vi "ProcessManager.vi"() -> ()   [LabVIEW 2019]
doc: "Fonction :\n\nCe modèle peut être intégré très facilement à un subpannel à l'aide des fonctions de la palette Code Template >> Dynamic VI and Subpanel de la VIBOX"
panel:
  out "data":string[][](array[string])=[["1", "芯轴分总成磨合台"], ["2", "上管柱组件装配"], ["3", "上管柱上转向轴合成"], ["4", "滑移力检测"], ["5", "芯轴分总成NVH"], ["6", "上转向轴组件装配"], ["7", "上下管柱总成装配"], ["8", "滑移力复检"], ["9", "最终性能试验台"], ["10", "传感器对中台"], ["11", "电机装配"], ["12", "中间轴装配"], ["13", "GP12（340）"], ["14", "ECU装配"], ["22", "激光打标机"], ["26", "调节机构检测"], ["29", "调节机构装配"]]
  out "ALL_DEVICE":string[](array[string])=["芯轴分总成磨合台", "上管柱组件装配", "上管柱上转向轴合成", "滑移力检测", "芯轴分总成NVH", "上转向轴组件装配", "上下管柱总成装配", "滑移力复检", "最终性能试验台", "传感器对中台", "电机装配", "中间轴装配", "GP12（340）", "ECU装配", "激光打标机", "调节机构检测", "调节机构装配"]
  out "Stop<user event>":refnum<user-event>
  in  "保存按钮":bool
  in  "产品型号":u16(ring) caption="Enum 3" items=[""=0, "R092B"=8, "R128"=1, "R527"=4, "R538"=5, "R563A"=9, "R563X"=7, "R567X"=6, "R92A"=3]
  in  "工位名称":i32(listbox)
  in  "产品工艺":string(tree)
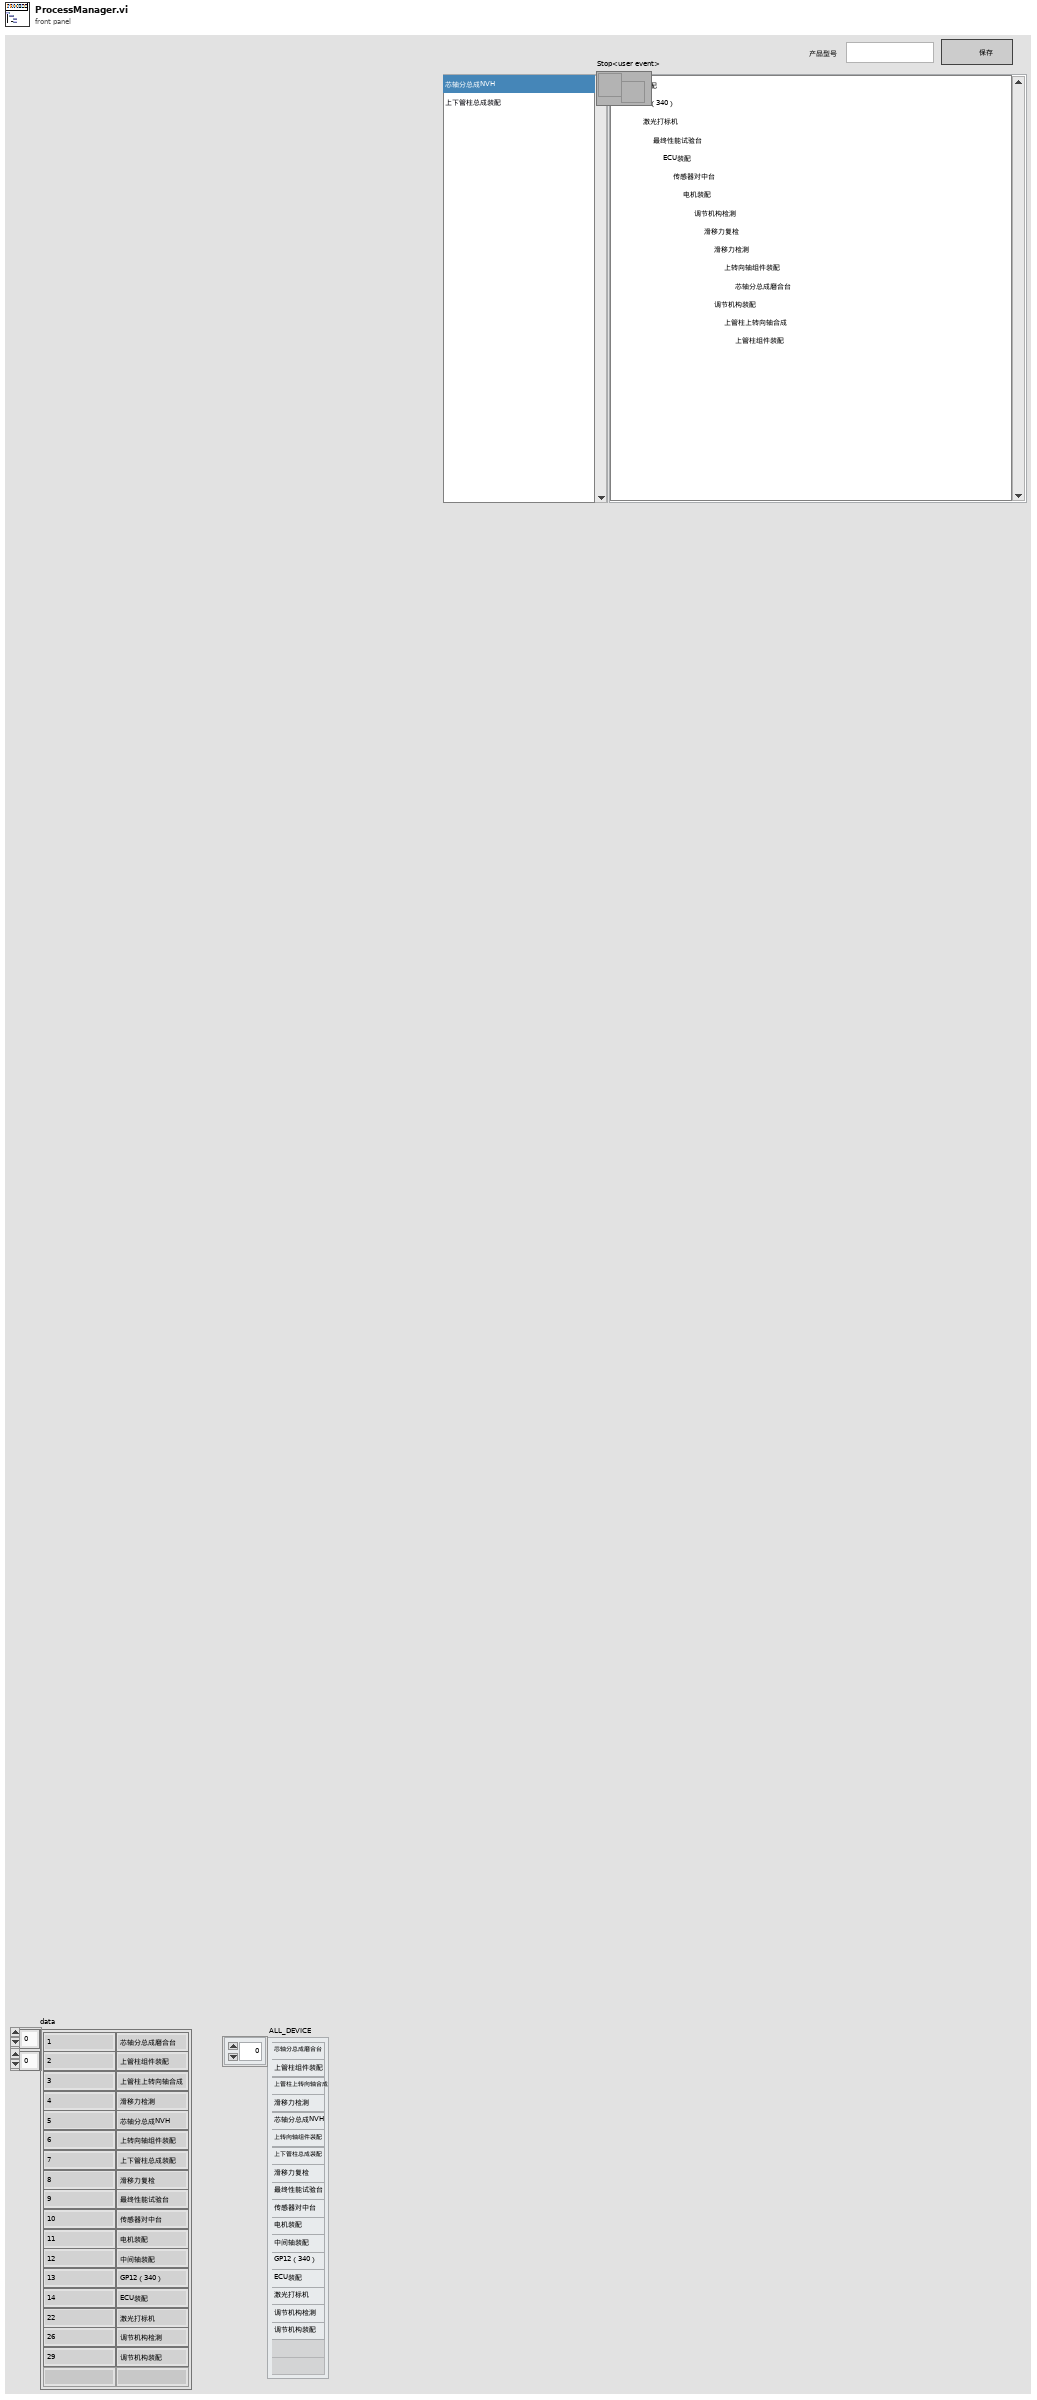
[diagram p1: front panel]
types:
  T1 = cluster{"data name":string, "drag data":variant}[]
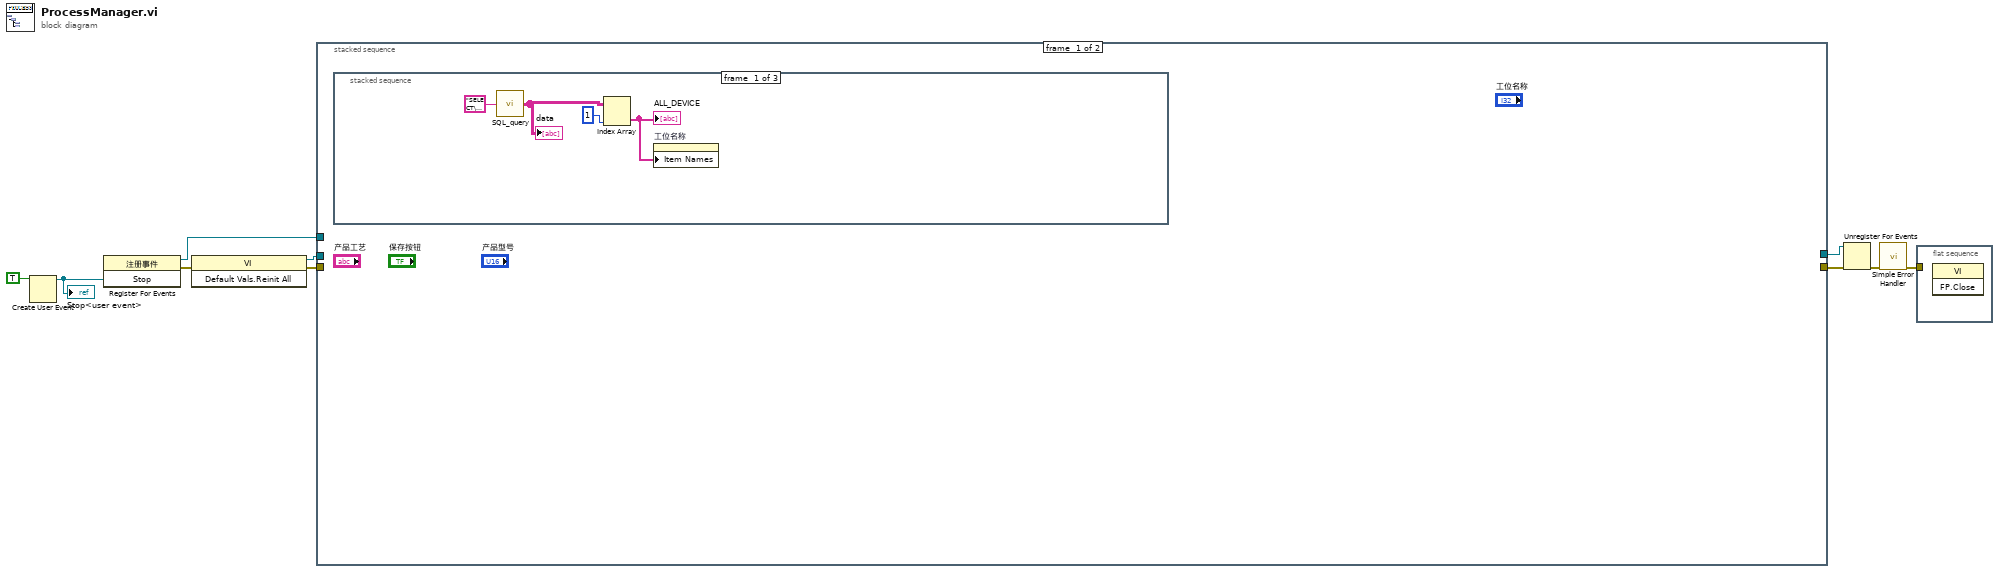
[diagram p0: block diagram]
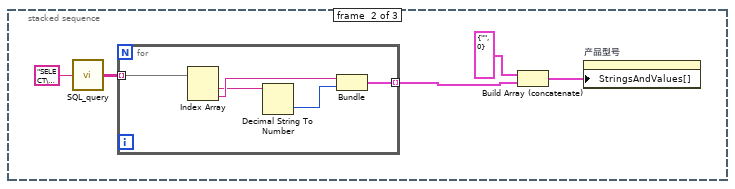
[diagram p2: hidden frame]
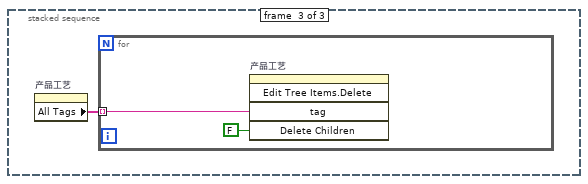
[diagram p3: hidden frame]
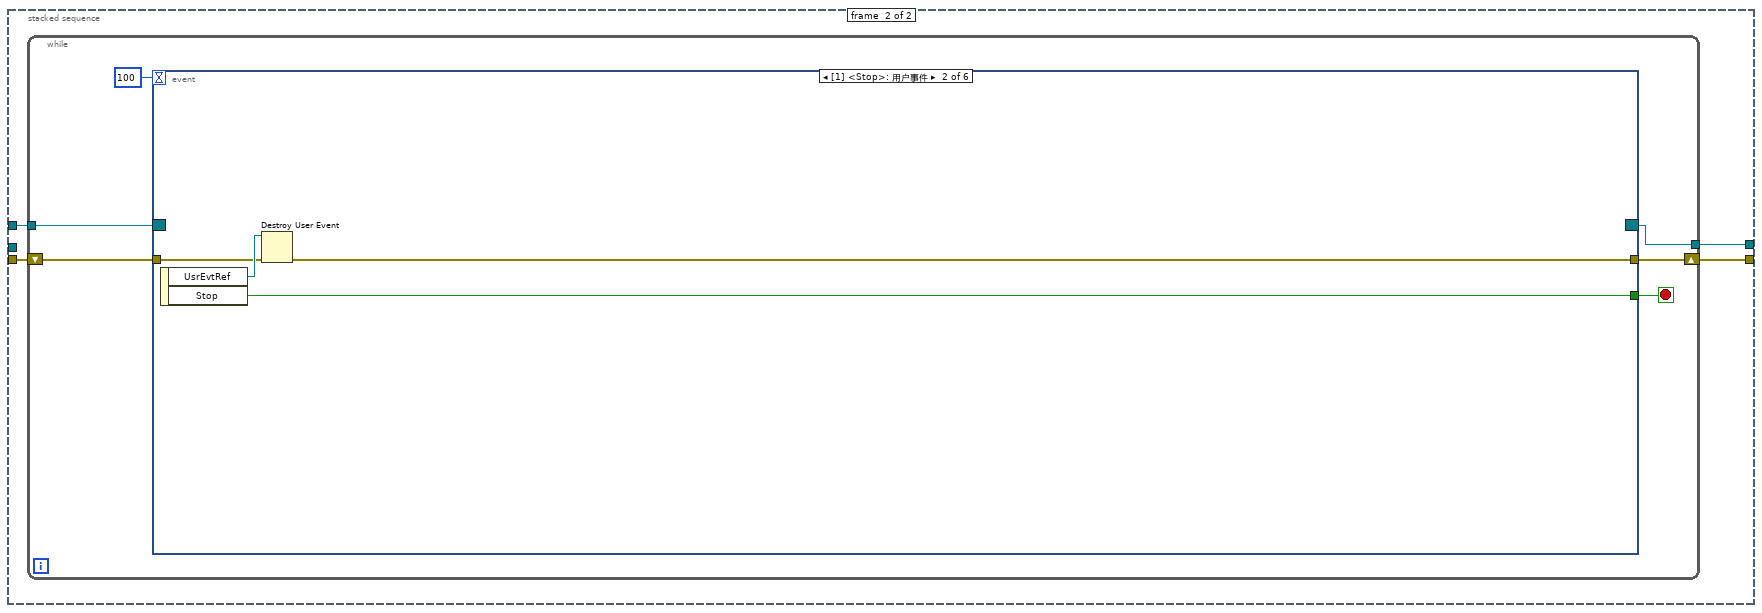
[diagram p4: hidden frame]
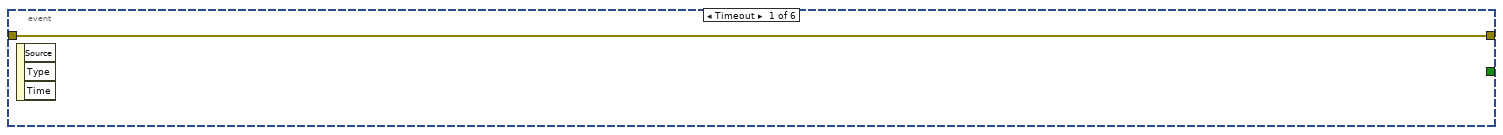
[diagram p5: hidden frame]
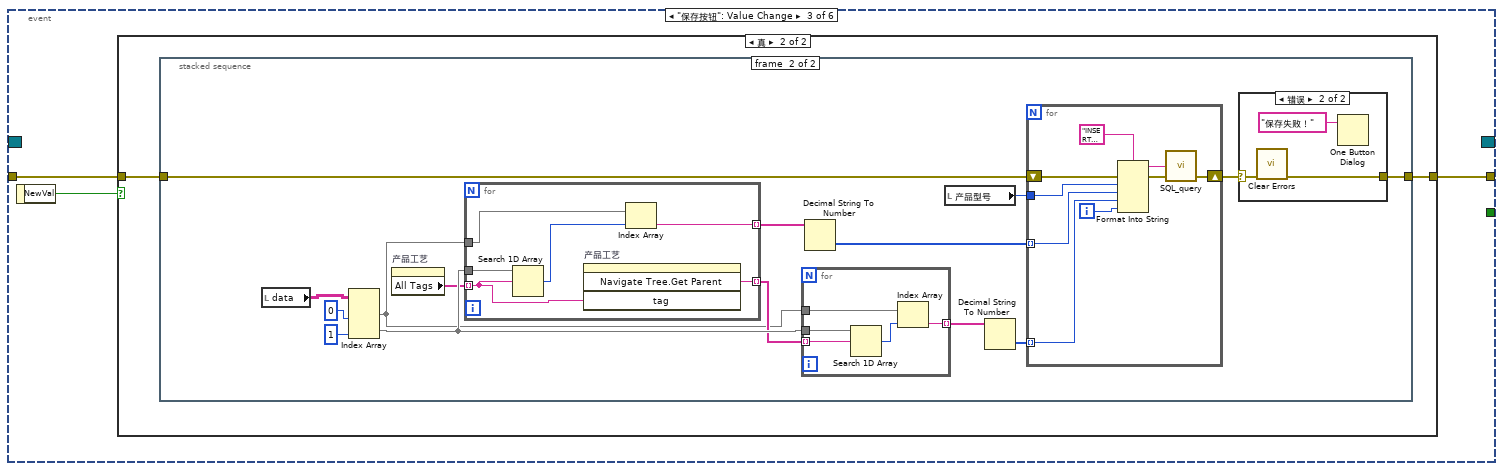
[diagram p6: hidden frame]
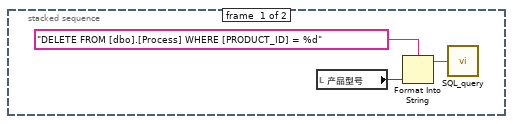
[diagram p8: hidden frame]
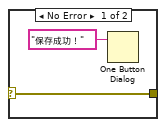
[diagram p9: hidden frame]
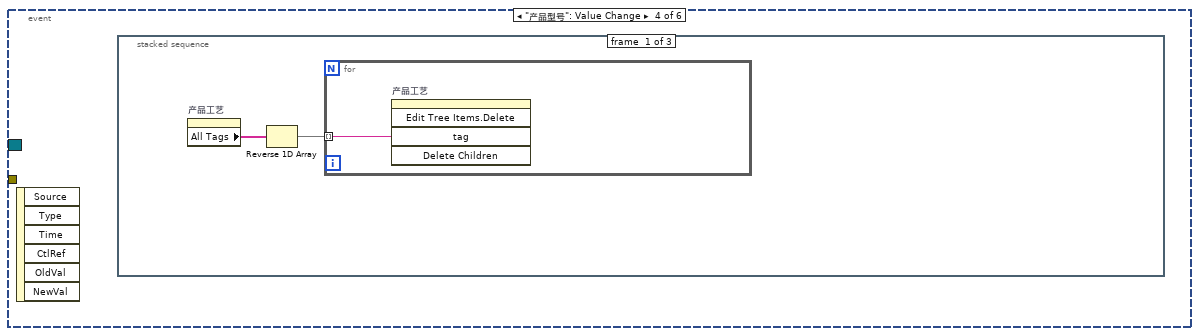
[diagram p10: hidden frame]
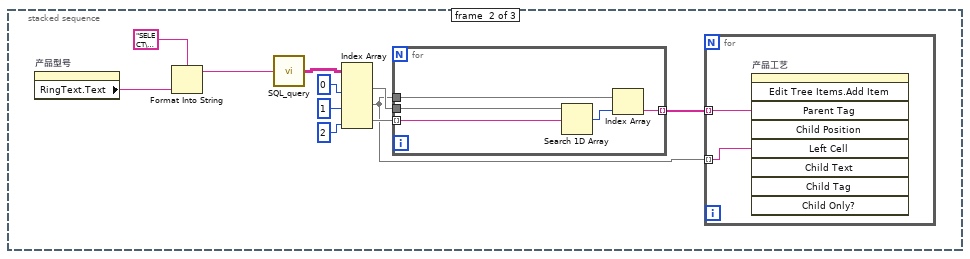
[diagram p11: hidden frame]
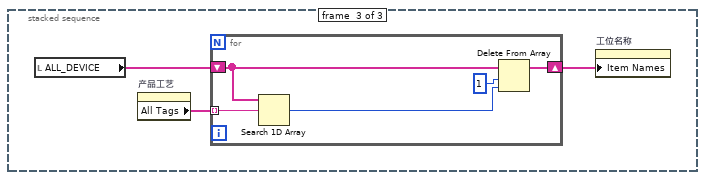
[diagram p12: hidden frame]
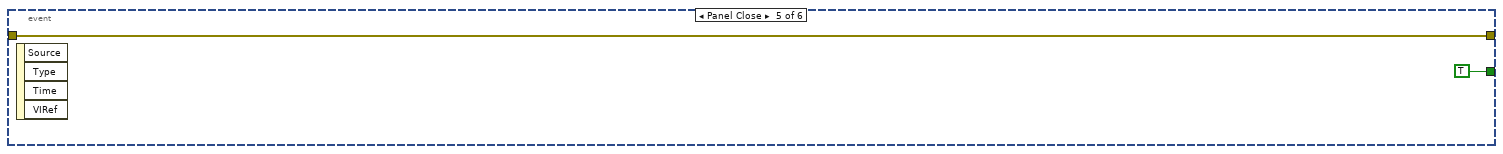
[diagram p13: hidden frame]
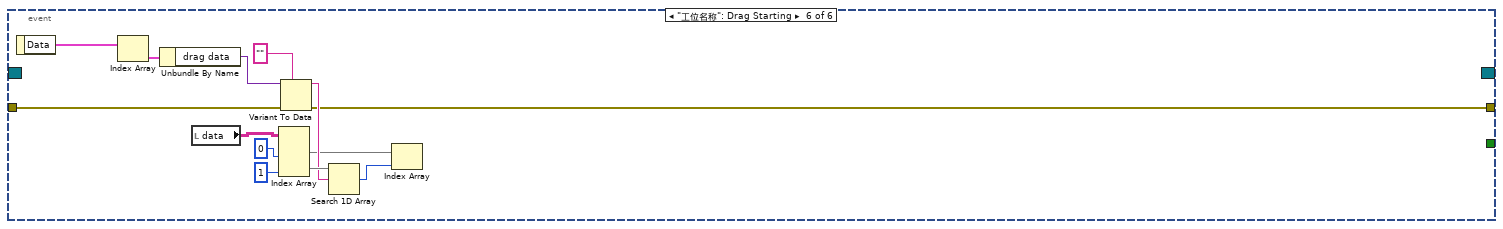
[diagram p14: hidden frame]
diagram:
  n1 = Create User Event(user event datatype=TRUE ("Stop")) -> (user event=w10:refnum<user-event>)  [unwired: 1 in, 1 out]
  "Stop<user event>" <- w10
  n2 = register-events(w10) -> (reference out=w6:refnum<event-registration>, error out=w7:errorcluster)  [unwired: 2 in]
  n3 = invoke class="VI" method="Default Vals.Reinit All"(error in=w7) -> (reference out=w8:refnum<vi>, error out=w5:errorcluster)  [unwired: 2 in, 1 out]
  n4 = stacked-sequence {
    tunnel: w8 -> [_ _]
    tunnel: w6 -> [_ w31]
    tunnel: w5 -> [_ w30]
    tunnel: [_ w28] -> w2
    tunnel: [_ w29] -> w1
    frame #0 {
      n5 = stacked-sequence {
        frame #0 {
          n6 = call "SQL_query.vi"("SQL query"="SELECT\ndbo.Device.DEVICE_ID,\ndbo.Device.DEVICE_NAME\n\nFROM\ndbo.Device\n") -> ("data"=w14:string[][])  [unwired: 2 in, 2 out]
          "data" <- w14
          n7 = Index Array(array=w14, index (col)=1 ("禁用的索引 (列)")) -> (element=w11:string[])  [unwired: 1 in]
          "ALL_DEVICE" <- w11
          n8 = property on="工位名称" class="LstBox (严格)"("Item Names"=w11) -> ()  [unwired: 2 in, 2 out]
        }
        frame #1 {
          n9 = call "SQL_query.vi"("SQL query"="SELECT\ndbo.Product.PRODUCT_ID,\ndbo.Product.PRODUCT_NAME\n\nFROM\ndbo.Product\n") -> ("data"=w18:string[][])  [unwired: 2 in, 2 out]
          n10 = for {
            tunnel: w18 -> [w24] mode=indexing
            tunnel: [w22] -> w19 mode=indexing
            n11 = Index Array(array=w24) -> (element #1=w21:string, element #2=w23:string)  [unwired: 2 in]
            n12 = Decimal String To Number(string=w21) -> (number=w20:i32)  [unwired: 2 in, 1 out]
            n13 = Bundle(w23, w20) -> (w22:cluster{string, i32})  [unwired: 1 in]
          }
          n14 = Build Array (concatenate)(cluster{string, i32} {"", 0}, w19) -> (w15:cluster{string, i32}[])
          n15 = property on="产品型号" class="Ring (严格)"("StringsAndValues[]"=w15) -> ()  [unwired: 2 in, 2 out]
        }
        frame #2 {
          n16 = property on="产品工艺" class="Tree (严格)"() -> ("All Tags"=w25:string[])  [unwired: 2 in, 2 out]
          n17 = for {
            tunnel: w25 -> [w27] mode=indexing
            n18 = invoke on="产品工艺" class="Tree (严格)" method="Edit Tree Items.Delete"("tag"=w27, "Delete Children"=FALSE ("删除子项？")) -> ()  [unwired: 3 in, 5 out]
          }
        }
      }
    }
    frame #1 {
      n19 = while {
        tunnel: w31 -> [w35]
        tunnel: [w32] -> w29
        shift-right: [w33] -> w28
        shift-left: w30 -> [w34]
        stop <- w37 stop-if-true
        n20 = event shown="[1] <Stop>: 用户事件" {
          selector: w35 -> [_ _ _ _ _ _]
          dyn-events: [_ _ _ _ _ _] -> w32
          timeout: 100 -> [_ _ _ _ _ _]
          tunnel: [_ w40 _ _ TRUE _] -> w37
          tunnel: w34 -> [w38 w41 w44 _ w121 w124]
          tunnel: [w38 w39 w43 _ w121 w123] -> w33
          event Timeout {
            n21 = event-data() -> ()  [unwired: 1 in, 3 out]
          }
          event User Event {
            n22 = event-data() -> ("UsrEvtRef"=w42:refnum<user-event>, "Stop"=w40:bool)  [unwired: 1 in]
            n23 = Destroy User Event(user event=w42, error in=w41) -> (error out=w39:errorcluster)
          }
          event "保存按钮": Value Change {
            n24 = event-data() -> ("NewVal"=w45:bool)  [unwired: 1 in]
            n25 = case shown="真" w45 {
              tunnel: w44 -> [w46 w48]
              tunnel: [w46 w47] -> w43
              frame False {
              }
              frame True {
                n26 = stacked-sequence {
                  tunnel: w48 -> [_ w53]
                  tunnel: [_ w52] -> w47
                  frame #0 {
                    n27 = local read "产品型号"() -> (w50:u16)
                    n28 = Format Into String(format string="DELETE FROM [dbo].[Process] WHERE [PRODUCT_ID] = %d", w50) -> (resulting string=w49:string)  [unwired: 2 in, 1 out]
                    n29 = call "SQL_query.vi"("SQL query"=w49) -> ()  [unwired: 2 in, 3 out]
                  }
                  frame #1 {
                    n30 = local read "data"() -> (w66:string[][])
                    n31 = Index Array(array=w66, index (col) #1=0 ("禁用的索引 (列)"), index (col) #2=1 ("索引 (列)")) -> (element #1=w63:string[], element #2=w65:string[])  [unwired: 2 in]
                    n32 = property on="产品工艺" class="Tree (严格)"() -> ("All Tags"=w54:string[])  [unwired: 2 in, 2 out]
                    n33 = for {
                      tunnel: w54 -> [w87] mode=indexing
                      tunnel: [w86] -> w64 mode=indexing
                      tunnel: w63 -> [w90]
                      tunnel: w65 -> [w91]
                      tunnel: [w88] -> w59 mode=indexing
                      n34 = Search 1D Array(1D array=w91, element=w87) -> (index of element=w89:i32)  [unwired: 1 in]
                      n35 = invoke on="产品工艺" class="Tree (严格)" method="Navigate Tree.Get Parent"("tag"=w87) -> ("Navigate Tree:Get Parent"=w86:string)  [unwired: 3 in, 3 out]
                      n36 = Index Array(array=w90, index=w89) -> (element=w88:string)
                    }
                    n37 = for {
                      tunnel: w65 -> [w84]
                      tunnel: w64 -> [w83] mode=indexing
                      tunnel: w63 -> [w82]
                      tunnel: [w81] -> w60 mode=indexing
                      n38 = Search 1D Array(1D array=w84, element=w83) -> (index of element=w85:i32)  [unwired: 1 in]
                      n39 = Index Array(array=w82, index=w85) -> (element=w81:string)
                    }
                    n40 = Decimal String To Number(string=w59) -> (number=w56:i32[])  [unwired: 2 in, 1 out]
                    n41 = local read "产品型号"() -> (w58:u16)
                    n42 = Decimal String To Number(string=w60) -> (number=w57:i32[])  [unwired: 2 in, 1 out]
                    n43 = for {
                      tunnel: w57 -> [w79] mode=indexing
                      tunnel: w56 -> [w78] mode=indexing
                      tunnel: w58 -> [w80]
                      shift-right: [w74] -> w55
                      shift-left: w53 -> [w73]
                      i -> [w75]
                      n44 = Format Into String(format string="INSERT INTO dbo.Process ( PRODUCT_ID, DEVICE_ID, PARENT_ID,LABVIEW_ID )\nVALUES\n\t(\n\t\t%d,\n\t\t%d,\n\t\t\t%d,\n%d)" ("格式字符串"), error in=w73, w80, w78, w79, w75) -> (resulting string=w77:string, error out=w72:errorcluster)  [unwired: 1 in]
                      n45 = call "SQL_query.vi"("error in (no error)"=w72, "SQL query"=w77) -> ("error out"=w74:errorcluster)  [unwired: 1 in, 2 out]
                    }
                    n46 = case shown="错误" w55 {
                      selector: w55 -> [w67 w69]
                      tunnel: [w67 w70] -> w52
                      frame No Error {
                        n47 = One Button Dialog(message="保存成功！" ("消息")) -> ()  [unwired: 1 in, 1 out]
                      }
                      frame Error {
                        n48 = call <vilib>:"Clear Errors.vi"("error in (no error)"=w69) -> ("error out"=w70:errorcluster)  [unwired: 5 in, 1 out]
                        n49 = One Button Dialog(message="保存失败！" ("消息")) -> ()  [unwired: 1 in, 1 out]
                      }
                    }
                  }
                }
              }
            }
          }
          event "产品型号": Value Change {
            n50 = event-data() -> ()  [unwired: 1 in, 6 out]
            n51 = stacked-sequence {
              frame #0 {
                n52 = property on="产品工艺" class="Tree (严格)"() -> ("All Tags"=w92:string[])  [unwired: 2 in, 2 out]
                n53 = Reverse 1D Array(array=w92) -> (reversed array=w93:string[])
                n54 = for {
                  tunnel: w93 -> [w94] mode=indexing
                  n55 = invoke on="产品工艺" class="Tree (严格)" method="Edit Tree Items.Delete"("tag"=w94) -> ()  [unwired: 4 in, 5 out]
                }
              }
              frame #1 {
                n56 = property on="产品型号" class="Ring (严格)"() -> ("RingText.Text"=w95:string)  [unwired: 2 in, 2 out]
                n57 = Format Into String(format string="SELECT\ndbo.Process.DEVICE_ID,\ndbo.Device.DEVICE_NAME,\ndbo.Process.PARENT_ID\n\nFROM\ndbo.Process\nINNER JOIN dbo.Device ON dbo.Process.DEVICE_ID = dbo.Device.DEVICE_ID\nINNER JOIN dbo.Product ON dbo.Process.PRODUCT_ID = dbo.Product.PRODUCT_ID\nWHERE\ndbo.Product.PRODUCT_NAME = '%s'\nORDER BY\ndbo.Process.LABVIEW_ID ASC\n", w95) -> (resulting string=w99:string)  [unwired: 2 in, 1 out]
                n58 = call "SQL_query.vi"("SQL query"=w99) -> ("data"=w105:string[][])  [unwired: 2 in, 2 out]
                n59 = Index Array(array=w105, index (col) #1=0 ("禁用的索引 (列)"), index (col) #2=1 ("索引 (列)"), index (col) #3=2 ("索引 (列)")) -> (element #1=w100:string[], element #2=w96:string[], element #3=w101:string[])  [unwired: 3 in]
                n60 = for {
                  tunnel: w96 -> [w110]
                  tunnel: w101 -> [w111] mode=indexing
                  tunnel: w100 -> [w112]
                  tunnel: [w108] -> w97 mode=indexing
                  n61 = Search 1D Array(1D array=w112, element=w111) -> (index of element=w109:i32)  [unwired: 1 in]
                  n62 = Index Array(array=w110, index=w109) -> (element=w108:string)
                }
                n63 = for {
                  tunnel: w97 -> [w107] mode=indexing
                  tunnel: w96 -> [w106] mode=indexing
                  n64 = invoke on="产品工艺" class="Tree (严格)" method="Edit Tree Items.Add Item"("Parent Tag"=w107, "Left Cell"=w106) -> ()  [unwired: 7 in, 9 out]
                }
              }
              frame #2 {
                n65 = local read "ALL_DEVICE"() -> (w115:string[])
                n66 = property on="产品工艺" class="Tree (严格)"() -> ("All Tags"=w114:string[])  [unwired: 2 in, 2 out]
                n67 = for {
                  tunnel: w114 -> [w120] mode=indexing
                  shift-right: [w116] -> w113
                  shift-left: w115 -> [w119]
                  n68 = Search 1D Array(1D array=w119, element=w120) -> (index of element=w117:i32)  [unwired: 1 in]
                  n69 = Delete From Array(array=w119, length=1 ("长度"), index=w117) -> (array with subset deleted=w116:string[])  [unwired: 1 out]
                }
                n70 = property on="工位名称" class="LstBox (严格)"("Item Names"=w113) -> ()  [unwired: 2 in, 2 out]
              }
            }
          }
          event Panel Close {
            n71 = event-data() -> ()  [unwired: 1 in, 4 out]
          }
          event "工位名称": Drag Starting {
            n72 = event-data() -> ("Data"=w131:T1)  [unwired: 1 in]
            n73 = Index Array(array=w131) -> (element=w130:cluster{"data name":string, "drag data":variant})  [unwired: 1 in]
            n74 = Unbundle By Name(w130) -> ("drag data"=w129:variant)
            n75 = local read "data"() -> (w135:string[][])
            n76 = Index Array(array=w135, index (col) #1=0 ("禁用的索引 (列)"), index (col) #2=1 ("索引 (列)")) -> (element #1=w126:string[], element #2=w132:string[])  [unwired: 2 in]
            n77 = Variant To Data(error in=w124, type="", Variant=w129) -> (data=w127:string, error out=w123:errorcluster)
            n78 = Search 1D Array(1D array=w132, element=w127) -> (index of element=w125:i32)  [unwired: 1 in]
            n79 = Index Array(array=w126, index=w125) -> ()  [unwired: 1 out]
          }
        }
      }
    }
  }
  n80 = Unregister For Events(event registration refnum=w1, error in=w2) -> (error out=w3:errorcluster)
  n81 = call <vilib>:"Simple Error Handler.vi"("error in (no error)"=w3) -> ("error out"=w4:errorcluster)  [unwired: 1 in, 7 out]
  n82 = flat-sequence {
    tunnel: w4 -> [_]
    frame #0 {
      n83 = invoke class="VI" method="FP.Close"() -> ()  [unwired: 3 in, 3 out]
    }
  }
